vi "serial.vi"() -> ()   [LabVIEW 2012]
uses:
  <vilib>/Instr/_visa.llb/VISA Configure Serial Port (Instr).vi
panel:
  in  "Stop Button 2":bool
  in  "?":refnum<visa-resource-name>
  out "read buffer":string
  in  "write buffer":string
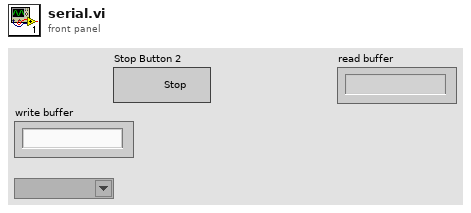
[diagram p1: front panel]
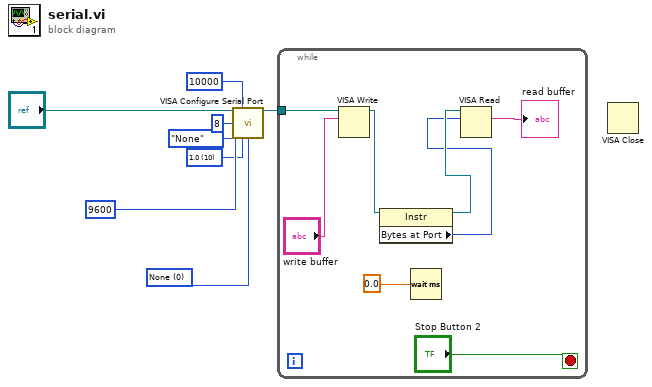
[diagram p0: block diagram]
diagram:
  w1 = u16 0 items=["None", "XON/XOFF", "RTS/CTS", "XON/XOFF & RTS/CTS", "DTR/DSR", "XON/XOFF & DTR/DSR"] ("flow control (0:none)")
  w2 = u16 10 items=["1.0"=10, "1.5"=15, "2.0"=20] ("stop bits (10: 1 bit)")
  n1 = call-poly "VISA Configure Serial Port"("VISA resource name"="?", "timeout (10sec)"=u32 10000, "baud rate (9600)"=u32 9600, "data bits (8)"=u16 8, "parity (0:none)"=enum16{"None", "Odd", "Even", "Mark", "Space"}."None", "stop bits (10: 1 bit)"=w2, "flow control (0:none)"=w1) -> ("VISA resource name out"=w8:refnum<visa-resource-name>)  [unwired: 7 in, 1 out]
  n2 = while {
    tunnel: w8 -> [w16]
    stop <- "Stop Button 2" stop-if-true
    n3 = VISA Write(VISA resource name=w16, write buffer="write buffer") -> (VISA resource name out=w15:refnum<visa-resource-name>)  [unwired: 1 in, 2 out]
    n4 = property class="Instr"(reference=w15) -> (reference out=w14:refnum<visa-resource-name>, "Bytes at Port"=w13:u32)  [unwired: 1 in, 1 out]
    n5 = Wait (ms)(milliseconds to wait=0.0) -> ()  [unwired: 1 out]
    n6 = VISA Read(VISA resource name=w14, byte count=w13) -> (read buffer=→"read buffer":string)  [unwired: 1 in, 3 out]
  }
  n7 = VISA Close() -> ()  [unwired: 2 in, 1 out]
